vi "Dipper Fridge Resistance Measurement 1.8.vi"() -> ()   [LabVIEW 2011]
panel:
  out "3He Pot":string
  in  "Sample Cell \nThermometer":bool
  out "Current Resistance":string
  in  "error in (no error) 3":errorcluster
  out "Sample Cell":string
  in  "error in (no error)":errorcluster
  in  "Heater option":string
  in  "Lakeshore":bool
  out "Sample Vs. Temp":cluster{dbl[], dbl[]}(graph)
  out "Warning":string="Can't be smaller than 1 s"
  in  "Time delay":u32
  in  "Timer":bool caption="Reset"
  out "Time Elapsed":string
  in  "Save":bool
  out "var":i32
  in  "error in (no error) 2":errorcluster
  out "Heater":bool
  in  "Heater":bool
  out "Boolean":bool
  in  "Power":bool
  in  "Date format (0)":enum16{"short", "long", "abbreviated"}(ring)
  out "size (in bytes)":i64
  out "Calibration":cluster{dbl[], dbl[]}(graph)
  in  "File Path":path
  out "current time":timestamp
  out "Number of Data points":i32
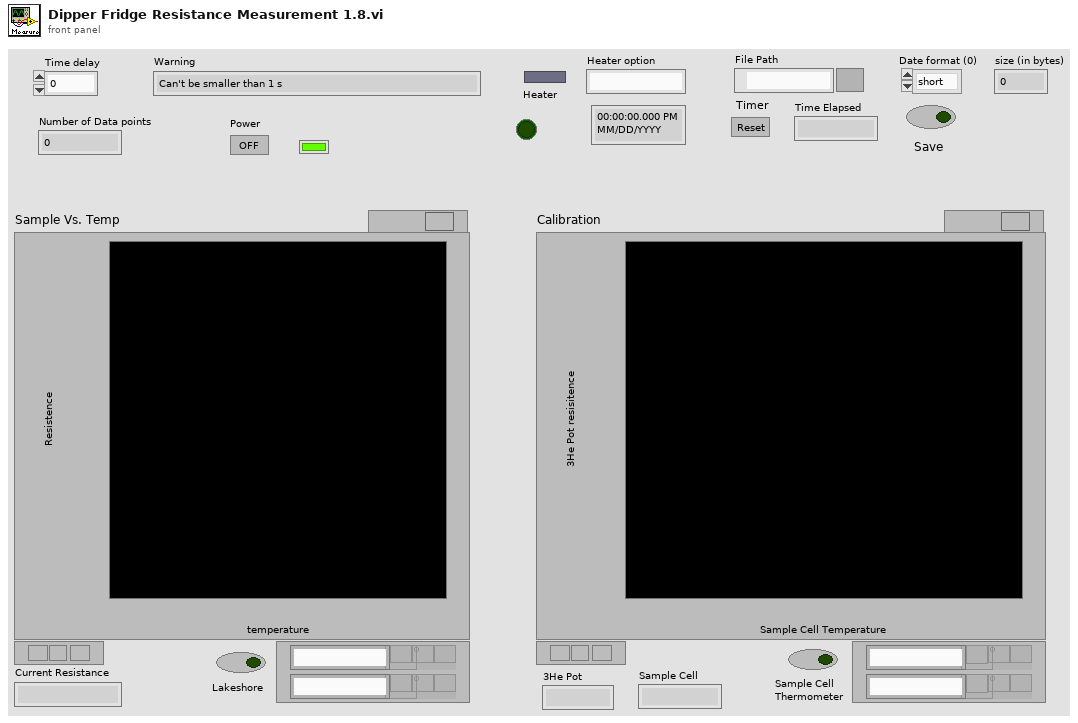
[diagram p1: front panel]
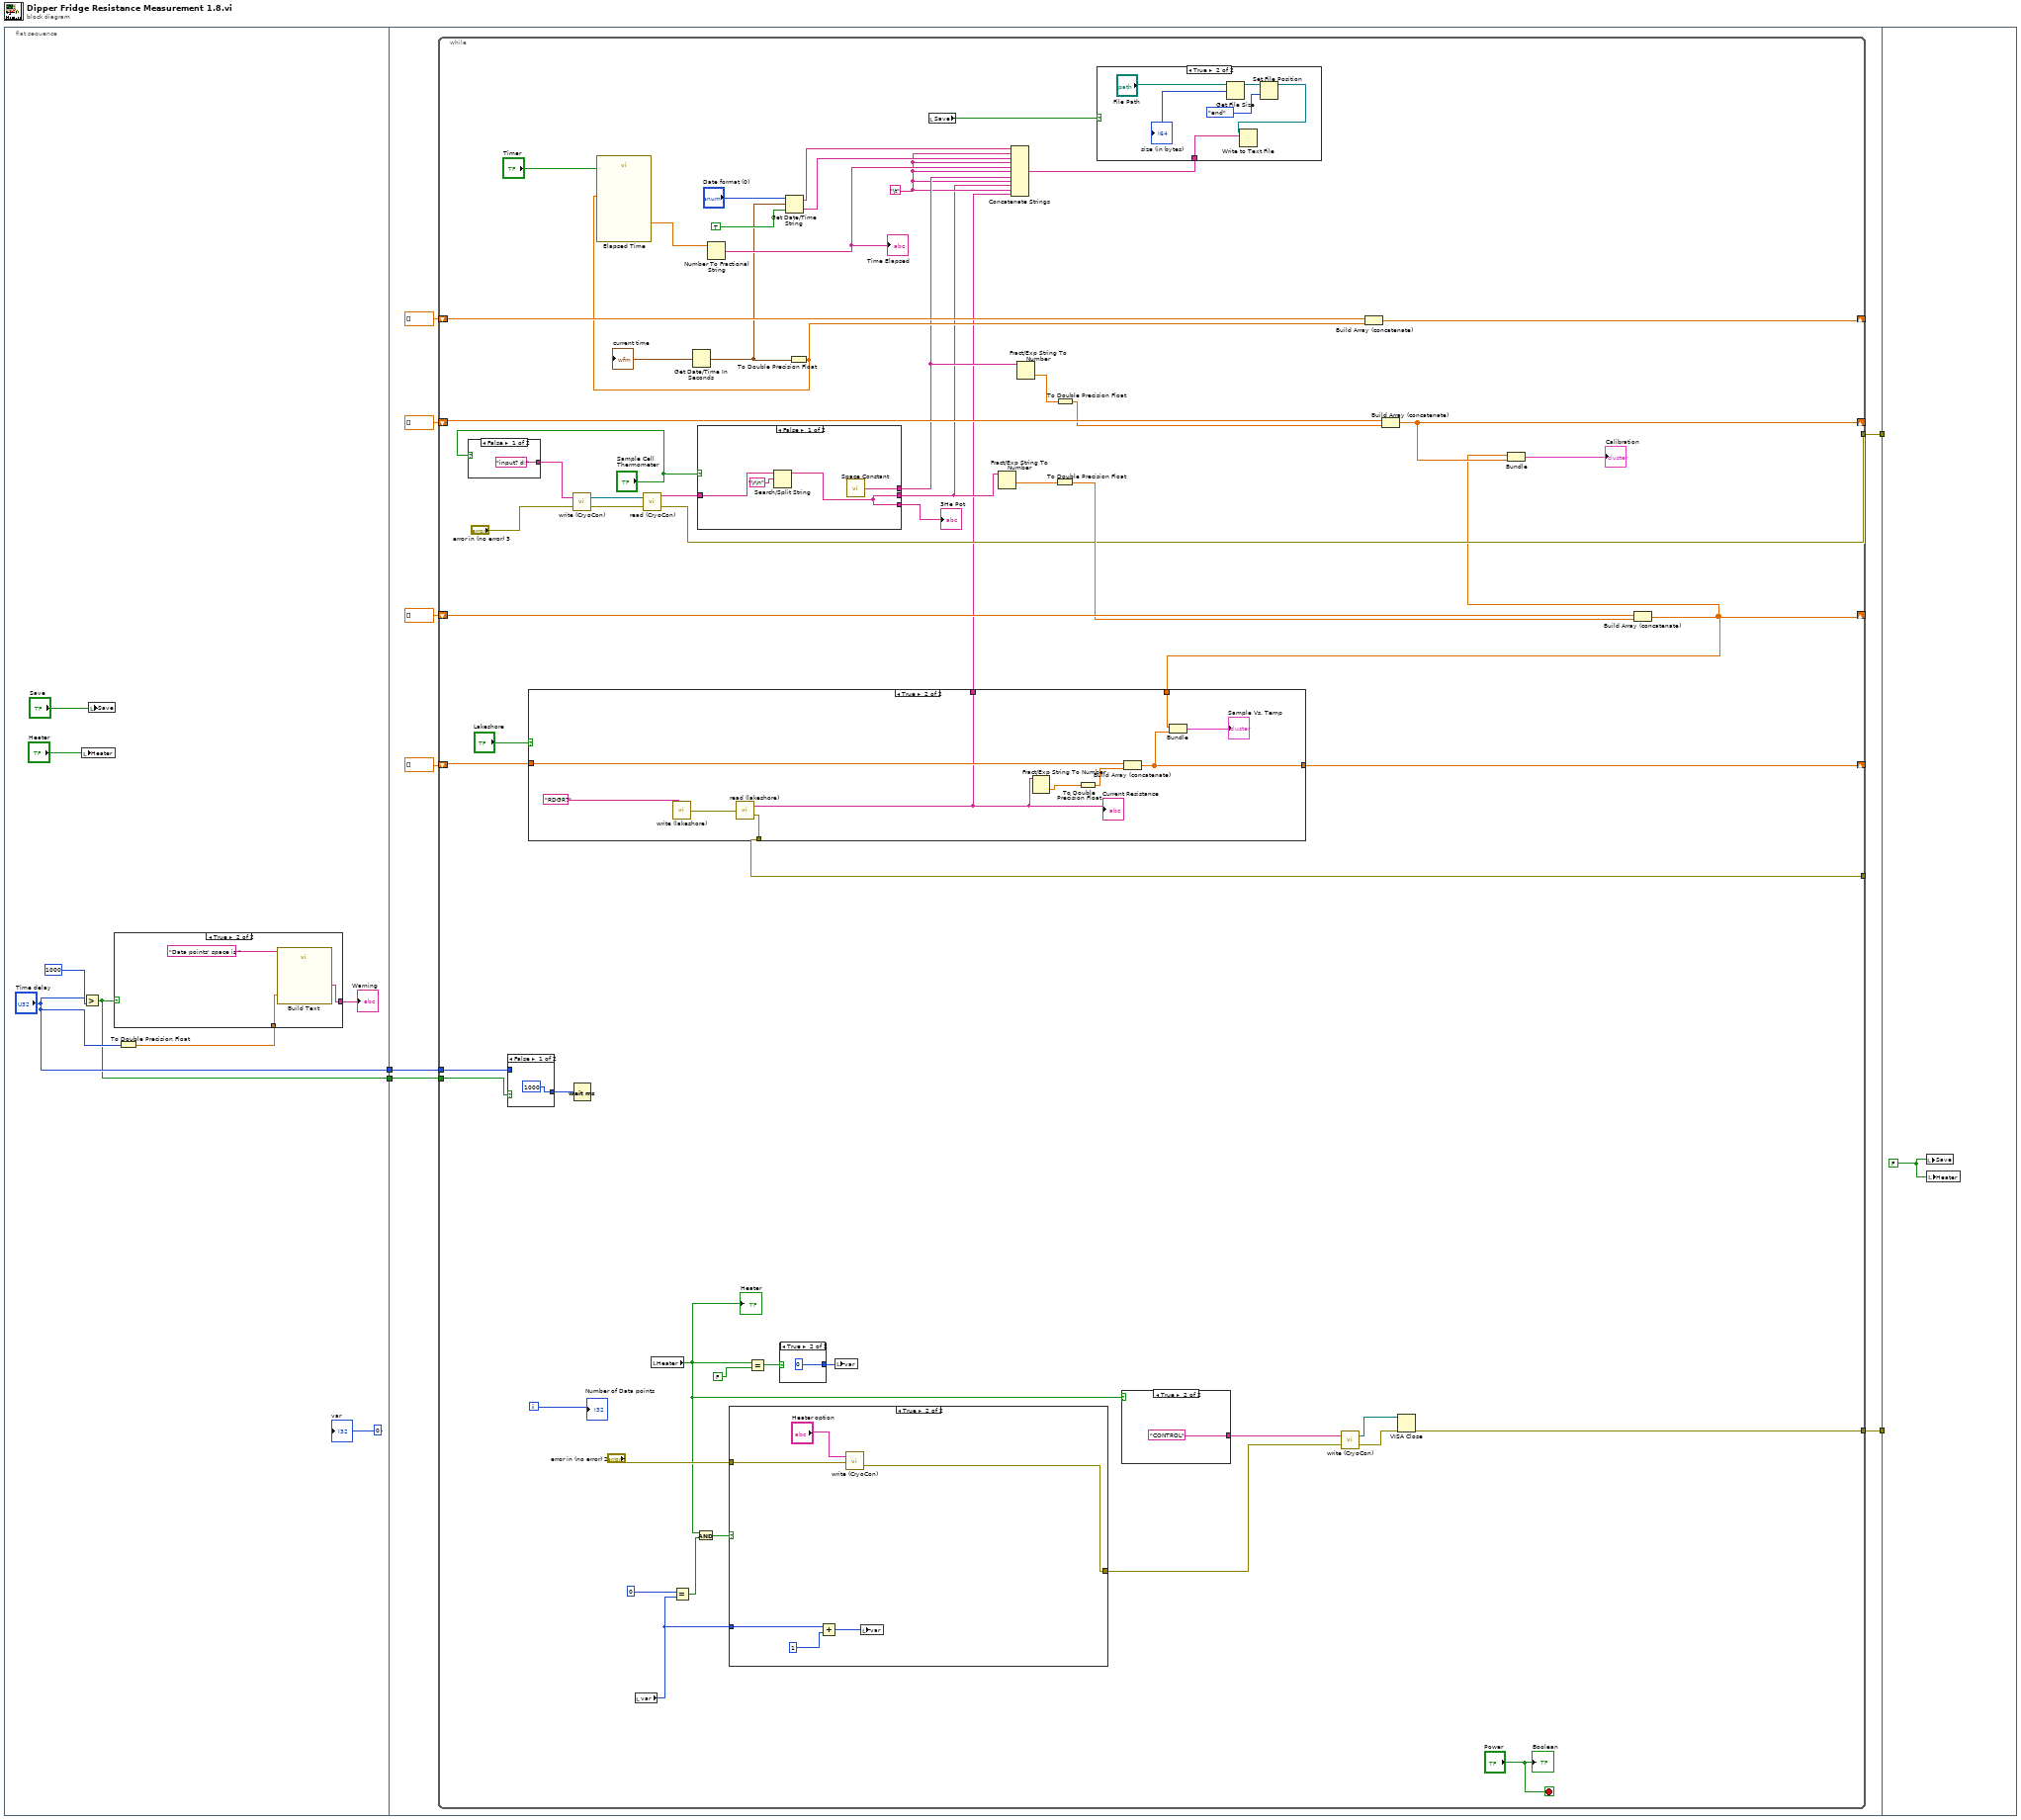
[diagram p0: block diagram]
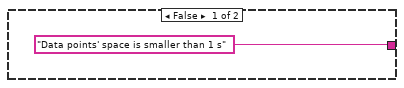
[diagram p2: hidden frame]
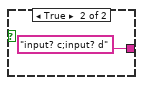
[diagram p3: hidden frame]
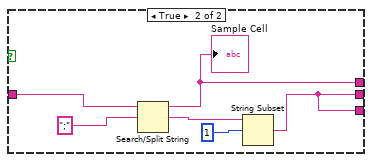
[diagram p4: hidden frame]
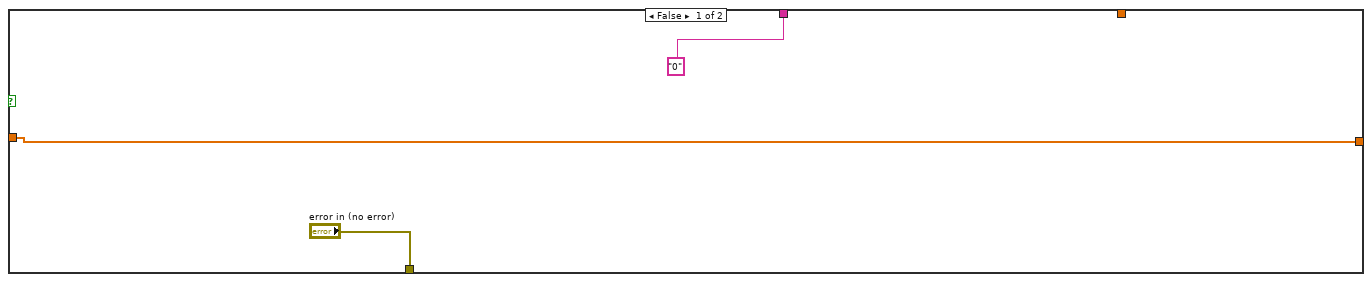
[diagram p5: hidden frame]
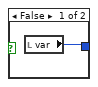
[diagram p7: hidden frame]
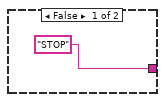
[diagram p9: hidden frame]
diagram:
  n1 = flat-sequence {
    tunnel: ["Time delay"] -> w4
    tunnel: [w5] -> w3
    tunnel: w4 -> [w20]
    tunnel: w3 -> [w19]
    tunnel: [w18] -> w2
    tunnel: [w17] -> w1
    tunnel: w2 -> [_]
    tunnel: w1 -> [_]
    frame #0 {
      n2 = local write "Heater"("Heater") -> ()
      n3 = Greater?(x="Time delay", y=u32 1000 ("x")) -> (0:w5:bool)
      n4 = local write "Save"("Save") -> ()
      n5 = To Double Precision Float(number="Time delay") -> (double precision float=w7:dbl)
      n6 = case shown="True" w5 {
        tunnel: w7 -> [_ w14]
        tunnel: ["Data points' space is smaller than 1 s" w16] -> w8
        frame False {
        }
        frame True {
          n7 = call "Build Text"("Beginning Text"="Data points' space is ", "Y"=w14) -> ("Result"=w16:string)  [unwired: 12 in, 1 out]
        }
      }
      "Warning" <- w8
      "var" <- 0 ("var")
    }
    frame #1 {
      n8 = while {
        tunnel: [w81] -> _
        shift-right: [w48] -> _
        shift-left: dbl[] [] -> [w78]
        shift-right: [w43] -> _
        shift-left: dbl[] [] -> [w75]
        shift-right: [w47] -> _
        shift-left: dbl[] [] -> [w53]
        shift-right: [w33] -> _
        shift-left: dbl[] [] -> [w52]
        tunnel: w20 -> [w49]
        tunnel: w19 -> [w50]
        tunnel: [w38] -> w18
        tunnel: [w34] -> w17
        i -> [w80]
        stop <- "Power" stop-if-true
        w27 = "\t"
        n9 = case shown="False" "Sample Cell \nThermometer" {
          tunnel: ["input? d;" "input? c;input? d"] -> w31
          frame False {
          }
          frame True {
          }
        }
        n10 = case shown="False" w50 {
          tunnel: [1000 w108] -> w51
          tunnel: w49 -> [_ w108]
          frame False {
          }
          frame True {
          }
        }
        n11 = call "write (CryoCon).vi"("error in (no error)"="error in (no error) 3", "write buffer"=w31) -> ("error out"=w37:errorcluster, "VISA resource name out"=w32:refnum<visa-resource-name>)
        n12 = Wait (ms)(milliseconds to wait=w51) -> ()  [unwired: 1 out]
        n13 = local read "var"() -> (w70:i32)
        n14 = call "read (CryoCon).vi"("error in (no error)"=w37, "VISA resource name"=w32) -> ("error out"=w38:errorcluster, "read buffer"=w39:string)
        n15 = local read "Heater"() -> (w61:bool)
        "Heater" <- w61
        n16 = Equal?(x=0, y=w70) -> (x = y?=w68:bool)
        n17 = Get Date/Time In Seconds() -> (seconds since 1Jan1904=w59:timestamp)
        "current time" <- w59
        n18 = And(x=w61, y=w68) -> (x .and. y?=w67:bool)
        n19 = case shown="False" "Sample Cell \nThermometer" {
          tunnel: w39 -> [w86 w90]
          tunnel: [w84 w88] -> w26
          tunnel: [w87 w89] -> w29
          tunnel: [w84 w88] -> w28
          frame False {
            n20 = Search/Split String(string=w86, search string/char (-)="\r\n") -> (substring before match=w84:string)  [unwired: 1 in, 2 out]
            n21 = call <vilib>:"Space Constant.vi"() -> ("String"=w87:string)
          }
          frame True {
            n22 = Search/Split String(string=w90, search string/char (-)=";") -> (substring before match=w89:string, match + rest of string=w92:string)  [unwired: 1 in, 1 out]
            "Sample Cell" <- w89
            n23 = String Subset(string=w92, offset (0)=1) -> (substring=w88:string)  [unwired: 1 in]
          }
        }
        "3He Pot" <- w28
        n24 = case shown="True" w67 {
          tunnel: [w111 w112] -> w66
          tunnel: "error in (no error) 2" -> [w111 w114]
          tunnel: w70 -> [_ w117]
          frame False {
          }
          frame True {
            n25 = Add(x=w117, y=1) -> (x+y=w115:i32)
            n26 = call "write (CryoCon).vi"("error in (no error)"=w114, "write buffer"="Heater option") -> ("error out"=w112:errorcluster)  [unwired: 1 out]
            n27 = local write "var"(w115) -> ()
          }
        }
        n28 = Equal?(x=w61, y=FALSE ("Heater")) -> (x = y?=w63:bool)
        n29 = case shown="True" w63 {
          tunnel: [w109 0] -> w62
          frame False {
            n30 = local read "var"() -> (w109:i32)
          }
          frame True {
          }
        }
        n31 = Get Date/Time String(date format (0)="Date format (0)", seconds (now)=w59, want seconds? (F)=TRUE) -> (date string=w54:string, time string=w55:string)
        n32 = To Double Precision Float(number=w59) -> (double precision float=w57:dbl)
        n33 = call "Elapsed Time"("Reset"="Timer", "Set Start Time (s)"=w57) -> ("Elapsed Time (s)"=w58:dbl)  [unwired: 10 in, 7 out]
        n34 = Number To Fractional String(number=w58) -> (F-format string=w60:string)  [unwired: 3 in]
        "Time Elapsed" <- w60
        n35 = local write "var"(w62) -> ()
        n36 = local read "Save"() -> (w65:bool)
        n37 = Fract/Exp String To Number(string=w26) -> (number=w42:dbl)  [unwired: 3 in, 1 out]
        n38 = Fract/Exp String To Number(string=w29) -> (number=w46:dbl)  [unwired: 3 in, 1 out]
        n39 = To Double Precision Float(number=w42) -> (double precision float=w41:dbl)
        n40 = To Double Precision Float(number=w46) -> (double precision float=w45:dbl)
        n41 = case shown="True" w61 {
          tunnel: ["STOP" ("write buffer") "CONTROL" ("write buffer")] -> w72
          frame False {
          }
          frame True {
          }
        }
        n42 = call "write (CryoCon).vi"("error in (no error)"=w66, "write buffer"=w72) -> ("error out"=w35:errorcluster, "VISA resource name out"=w36:refnum<visa-resource-name>)
        n43 = Build Array (concatenate)(w78, w57) -> (w48:dbl[])
        n44 = Build Array (concatenate)(w75, w45) -> (w43:dbl[])
        n45 = VISA Close(VISA resource name=w36, error in (no error)=w35) -> (error out=w34:errorcluster)
        n46 = Build Array (concatenate)(w52, w41) -> (w33:dbl[])
        n47 = case shown="True" "Lakeshore" {
          tunnel: ["error in (no error)" w106] -> w81
          tunnel: w53 -> [w95 w103]
          tunnel: ["0" ("read buffer") w102] -> w25
          tunnel: [w95 w99] -> w47
          tunnel: w33 -> [_ w97]
          frame False {
          }
          frame True {
            n48 = call "write (lakeshore).vi"("write buffer"="RDGR?") -> ("error out"=w105:errorcluster)  [unwired: 1 in]
            n49 = call "read (lakeshore).vi"("error in (no error)"=w105) -> ("read buffer"=w102:string, "error out"=w106:errorcluster)
            "Current Resistance" <- w102
            n50 = Fract/Exp String To Number(string=w102) -> (number=w101:dbl)  [unwired: 3 in, 1 out]
            n51 = To Double Precision Float(number=w101) -> (double precision float=w100:dbl)
            n52 = Build Array (concatenate)(w103, w100) -> (w99:dbl[])
            n53 = Bundle(w97, w99) -> (→"Sample Vs. Temp":cluster{dbl[], dbl[]})  [unwired: 1 in]
          }
        }
        n54 = Concatenate Strings(w54, w27, w55, w27, w60, w27, w29, w27, w26, w27, w25) -> (w77:string)
        n55 = case shown="True" w65 {
          tunnel: w77 -> [_ w125]
          frame False {
          }
          frame True {
            n56 = Get File Size(file="File Path") -> (refnum out=w123:refnum<file>, size (in bytes)=→"size (in bytes)":i64)  [unwired: 1 in, 1 out]
            n57 = Set File Position(refnum=w123, from (0:start)=enum16{"start", "end", "current"}."end") -> (refnum out=w122:refnum<file>)  [unwired: 2 in, 1 out]
            n58 = Write to Text File(file (use dialog)=w122, text=w125) -> ()  [unwired: 2 in, 3 out]
          }
        }
        n59 = Bundle(w33, w43) -> (→"Calibration":cluster{dbl[], dbl[]})  [unwired: 1 in]
        "Number of Data points" <- w80
        "Boolean" <- "Power"
      }
    }
    frame #2 {
      w126 = FALSE ("Save")
      n60 = local write "Save"(w126) -> ()
      n61 = local write "Heater"(w126) -> ()
    }
  }
